vi "Enumerate Cameras.vi"(8 "error in":errorcluster, 11 "Data in":T1) -> (0 "error out":errorcluster, 3 "Data out":T1)   [LabVIEW 2020, in "AR Example.lvlib"]
uses:
  AR Example.lvlib
  Data.ctl
  g_ar_toolkit.capture/CameraManager/CameraManager.lvclass
  Tab Control.ctl
  State.ctl
  Global Events.ctl
  7a001a07-3868-4b83-bf2a-ac1a4e45c756.vi
  279f112d-e8f7-4047-9a36-8648f39be8ce.vi
  <vilib>/Comparison/Equal/Equal Functor/Equal Functor.lvclass
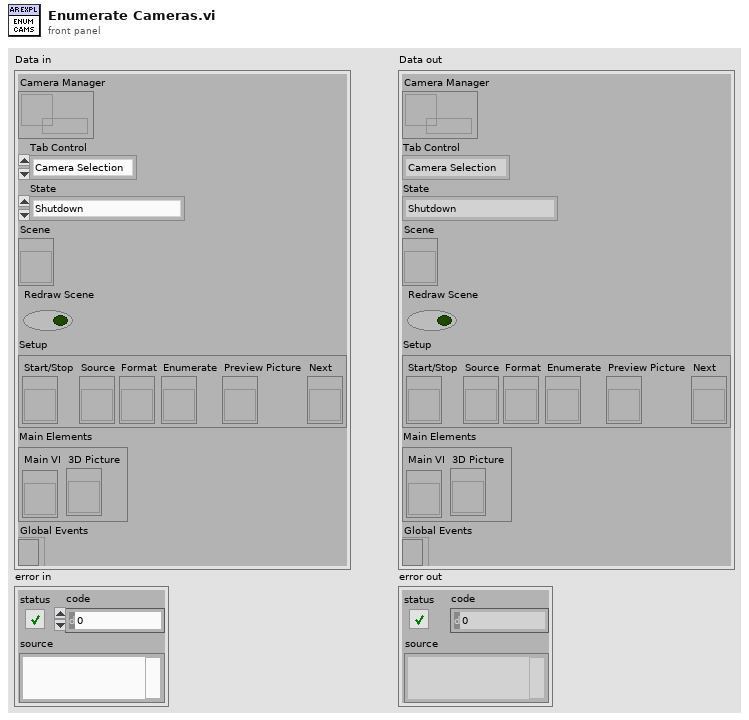
[diagram p1: front panel]
types:
  T1 = typedef "AR Example.lvlib/Data.ctl" = cluster{"Camera Manager":refnum<data-value>, "Tab Control":T2, "State":T3, "Scene":refnum<vi>, "Redraw Scene":bool, "Setup":cluster{"Start/Stop":refnum<vi>, "Source":refnum<vi>, "Format":refnum<vi>, "Enumerate":refnum<vi>, "Preview Picture":refnum<vi>, "Next":refnum<vi>}, "Main Elements":cluster{"Main VI":refnum<vi>, "3D Picture":refnum<vi>}, "Global Events":T4}
  T2 = typedef "AR Example.lvlib/Tab Control.ctl" = enum8{"Camera Selection"}
  T3 = typedef "AR Example.lvlib/State.ctl" = enum16{"Shutdown", "Initialize", "Select Camera"}
  T4 = typedef "AR Example.lvlib/Global Events.ctl" = refnum<event-registration>
  T5 = typedef "g_ar_toolkit.capture.lvlib/CameraManager.lvclass/Device Enumeration.ctl" = cluster{"Name":string, "Streams":set{T6}}
  T6 = typedef "g_ar_toolkit.capture.lvlib/CameraManager.lvclass/Stream Parameters.ctl" = cluster{"Width":u16, "Height":u16, "FPS":u8}
  T7 = enum8{"Enabled", "Disabled", "Disabled and Grayed Out"}
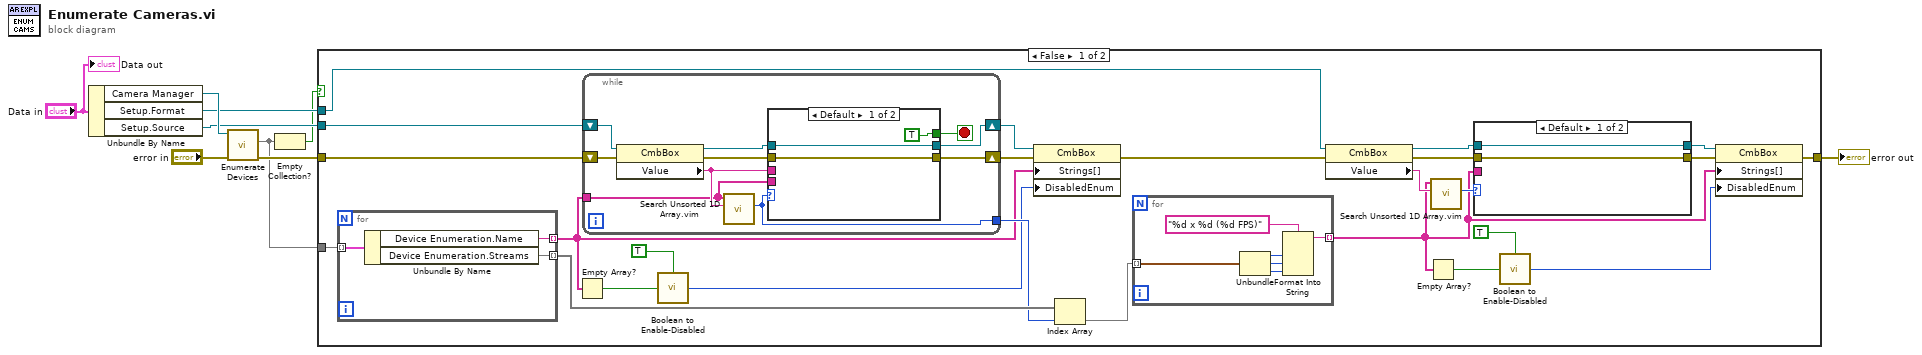
[diagram p0: block diagram]
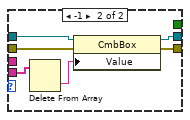
[diagram p2: hidden frame]
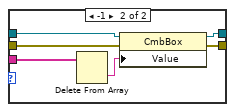
[diagram p3: hidden frame]
diagram:
  n1 = Unbundle By Name("Data in") -> ("Camera Manager"=w9:refnum<data-value>, "Setup.Format"=w8:refnum<vi>, "Setup.Source"=w7:refnum<vi>)
  n2 = call "Enumerate Devices.vi"("error in (no error)"="error in", "CameraManager"=w9) -> ("error out"=w5:errorcluster, "Devices"=w4:map{string, T5})  [unwired: 7 in, 1 out]
  n3 = Empty Collection?(1:w4) -> (0:w3:bool)
  n4 = case shown="False" w3 {
    tunnel: w8 -> [w17 _]
    tunnel: w5 -> [w28 w71]
    tunnel: w4 -> [w34 _]
    tunnel: w7 -> [w31 _]
    tunnel: [w33 w71] -> w2
    frame False {
      n5 = for {
        tunnel: w34 -> [w70] mode=indexing
        tunnel: [w69] -> w30 mode=indexing
        tunnel: [w68] -> w21 mode=indexing
        n6 = Unbundle By Name(w70) -> ("Device Enumeration.Name"=w68:string, "Device Enumeration.Streams"=w69:set{T6})
      }
      n7 = Empty Array?(array=w21) -> (empty?=w20:bool)
      n8 = while {
        tunnel: w21 -> [w38]
        tunnel: [w41] -> w27
        shift-right: [w37] -> w32
        shift-left: w28 -> [w43]
        shift-right: [w36] -> w25
        shift-left: w31 -> [w44]
        stop <- w35 stop-if-true
        n9 = property class="CmbBox"(reference=w44, error in=w43) -> (reference out=w40:refnum<vi>, error out=w39:errorcluster, "Value"=w42:string)
        n10 = call "Search Unsorted 1D Array.vim"("element"=w42, "unsorted 1D array"=w38) -> ("index of element"=w41:i32)  [unwired: 9 in]
        n11 = case shown="Default" w41 {
          tunnel: w38 -> [_ w53]
          tunnel: w42 -> [_ _]
          tunnel: [TRUE _] -> w35
          tunnel: w40 -> [w45 w52]
          tunnel: w39 -> [w46 w51]
          tunnel: [w46 w49] -> w37
          tunnel: [w45 w48] -> w36
          frame Default {
          }
          frame -1 {
            n12 = Delete From Array(array=w53) -> (deleted portion=w50:string)  [unwired: 2 in, 1 out]
            n13 = property class="CmbBox"(reference=w52, error in=w51, "Value"=w50) -> (reference out=w48:refnum<vi>, error out=w49:errorcluster)
          }
        }
      }
      n14 = call "Boolean to Enable-Disabled.vi"("Enabled?"=w20, "Invert?  (Default: False)"=TRUE) -> ("Disabled State"=w18:T7)
      n15 = property class="CmbBox"(reference=w25, error in=w32, "Strings[]"=w21, "DisabledEnum"=w18) -> (error out=w26:errorcluster)  [unwired: 1 out]
      n16 = Index Array(array=w30, index=w27) -> (element=w29:set{T6})
      n17 = for {
        tunnel: w29 -> [w67] mode=indexing
        tunnel: [w62] -> w10 mode=indexing
        n18 = Unbundle(w67) -> ("Width"=w66:u16, "Height"=w65:u16, "FPS"=w64:u8)
        n19 = Format Into String(format string="%d x %d (%d FPS)", w66, w65, w64) -> (resulting string=w62:string)  [unwired: 2 in, 1 out]
      }
      n20 = property class="CmbBox"(reference=w17, error in=w26) -> (reference out=w14:refnum<vi>, error out=w13:errorcluster, "Value"=w16:string)
      n21 = Empty Array?(array=w10) -> (empty?=w24:bool)
      n22 = call "Search Unsorted 1D Array.vim"("element"=w16, "unsorted 1D array"=w10) -> ("index of element"=w15:i32)  [unwired: 9 in]
      n23 = case shown="Default" w15 {
        tunnel: w14 -> [w55 w61]
        tunnel: w13 -> [w54 w60]
        tunnel: [w55 w59] -> w12
        tunnel: [w54 w58] -> w11
        tunnel: w10 -> [_ w57]
        frame Default {
        }
        frame -1 {
          n24 = Delete From Array(array=w57) -> (deleted portion=w56:string)  [unwired: 2 in, 1 out]
          n25 = property class="CmbBox"(reference=w61, error in=w60, "Value"=w56) -> (reference out=w59:refnum<vi>, error out=w58:errorcluster)
        }
      }
      n26 = call "Boolean to Enable-Disabled.vi"("Enabled?"=w24, "Invert?  (Default: False)"=TRUE) -> ("Disabled State"=w23:T7)
      n27 = property class="CmbBox"(reference=w12, error in=w11, "Strings[]"=w10, "DisabledEnum"=w23) -> (error out=w33:errorcluster)  [unwired: 1 out]
    }
    frame True {
    }
  }
  "error out" <- w2
  "Data out" <- "Data in"
